vi "Get Safety Config Path.vi"(8 "error in (no error)":errorcluster) -> (0 "error out":errorcluster, 3 "Safety Config path":path)   [LabVIEW 2018]
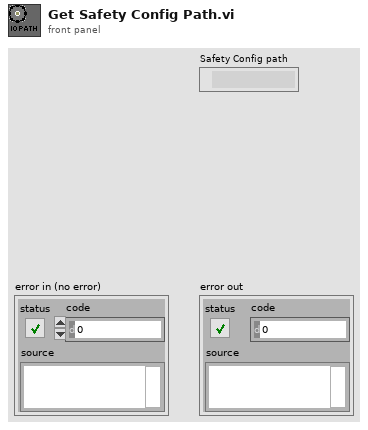
[diagram p1: front panel]
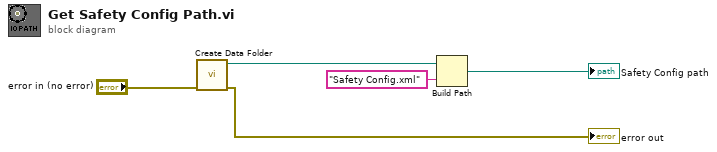
[diagram p0: block diagram]
diagram:
  n1 = call "Create Data Folder.vi"("error in (no error)"="error in (no error)") -> ("error out"=→"error out":errorcluster, "Data path"=w5:path)  [unwired: 9 in]
  n2 = Build Path(base path=w5, name or relative path="Safety Config.xml") -> (appended path=→"Safety Config path":path)
